vi "runnerFrontEnd.vi"(6 "ExperimentControlEvents":refnum<class "ExperimentControlEvents.lvclass">, 8 "error in (no error)":errorcluster, 9 "deviceDataBase":refnum<class "deviceDataBase.lvclass">, 10 "HWControllerEvents":refnum<class "HWControllerEvents.lvclass">, 11 "Views.lvlib:ExperimentControl.lvlib:ExperimentRunner in":refnum<class "ExperimentRunner.lvclass">) -> (0 "error out":errorcluster, 3 "Views.lvlib:ExperimentControl.lvlib:ExperimentRunner out":refnum<class "ExperimentRunner.lvclass">)   [LabVIEW 2011, in "Views.lvlib" / "ExperimentControl.lvlib" / "ExperimentRunner.lvclass"]
doc: "Experiment Runner Front End.\n\nThis is the user interface to control the expeirment. I.e. Run scripts and control the hardware state."
uses:
  ExperimentRunner.lvclass
  Hal/HWController/HWControllerEvents/HWControllerEvents.lvclass
  Tools/DatabaseHelpers/DbConnection/DeviceDataBase/deviceDataBase.lvclass
  Events/ExperimentControlEvents.lvclass
  ExperimentRunner.lvclass/ExperimentRunner.ctl
  CameraControlViewer/CameraControlViewer.lvclass
  Tools/SettingsProcessors/Compiler/Compiler.lvclass
  ScriptEditor/ScriptEditorV2/ScriptEditorV2.lvclass
  EventEditor/StaticOutputEditor/StaticOutputEditor.lvclass
  ScriptEditor/ScriptEdEvents/ScriptEdEvents.lvclass
  Tools/Filing/FileNeologist/FileNeologist.lvclass
  <vilib>/Utility/error.llb/DialogType.ctl
  Tools/DatabaseHelpers.lvlib
  Tools/Filing.lvlib
panel:
  in  "experimentFunction":enum16{"runListOnce", "loopOverList"}(ring)
  out "runningScriptName":string
  in  "HW Loop?":bool
  in  "refreshDatabase":bool
  in  "staticOutput":bool
  in  "stop":bool
  in  "runScript":bool
  in  "viewScript":bool
  in  "removePath":bool
  in  "addPath":bool
  out "status":T1(ring)
  in  "Listbox":i32(listbox)
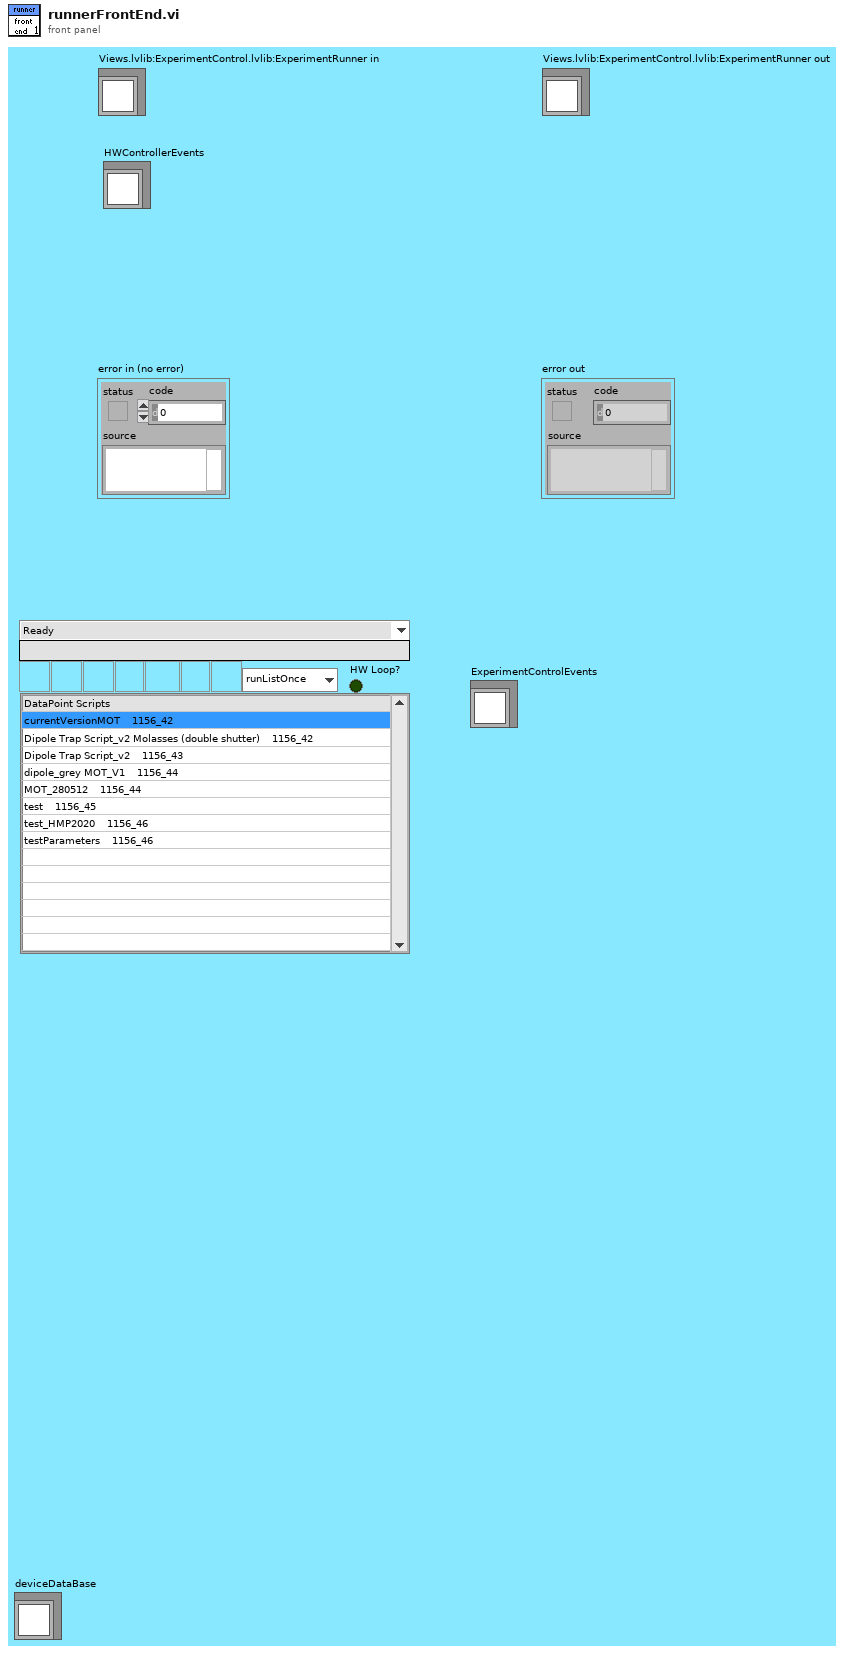
[diagram p1: front panel]
types:
  T1 = enum16{"Ready", "Compiling", "Configured", "Running", "Stopping", "Unresolved Error"}
  T2 = enum16{"start", "stop", "statusInquiry", "configure", "resetError", "resourcesInquiry", "reserveResources", "initialise", "resetAllChannels", "staticUpdate", "close", "HWStatus", "error", "resourcesAvailable", "resourcesReserved", "compilerError", "compiledScript", "compilingScript", "runScript", "configureCompiledScript"}
  T3 = enum16{"start", "stop", "statusInquiry", "configure", "resetError", "resourcesInquiry", "reserveResources", "initialise", "resetAllChannels", "staticUpdate", "close", "HWStatus", "error", "resourcesAvailable", "resourcesReserved"}
  T4 = enum16{"start", "stop", "statusInquiry", "configure", "resetError", "resourcesInquiry", "reserveResources", "initialise", "resetAllChannels", "staticUpdate", "close", "HWStatus", "error", "resourcesAvailable", "resourcesReserved", "compilerError", "compiledScript", "compilingScript", "runScript", "configureCompiledScript", "restartCompiler"}
  T5 = cluster{"incomingEventTypes":cluster{"start":cluster{"Boolean":bool}, "stop":cluster{"Boolean":bool}, "statusInquiry":cluster{"Boolean":bool}, "configure":cluster{"DPScriptPath":path, "TimeStamp":string, "HWLoop?":bool}, "resetError":cluster{"Boolean":bool}, "resourcesInquiry":cluster{"Boolean":bool}, "reserveResources":cluster{"HWList":string[]}, "initialise":cluster{"HWList":string[]}, "close":cluster{"Boolean":bool}, "resetAllChannels":cluster{"Boolean":bool}, "staticChannelUpdate":cluster{"channel_address":string, "calibratedValue":dbl}, "runScript":cluster{"DPScriptPath":path, "TimeStamp":string, "HWLoop?":bool}, "compilingScript":cluster{"Path":path}, "compiledScript":cluster{"Path":path, "timeCompileAt":string}, "compilerError":cluster{"Path":path}, "configureCompiledScript":cluster{"DPScriptPath":path, "TimeStamp":string, "HWLoop?":bool, "CompiledScript":cluster{"ScriptListCompiler.lvclass":refnum<class "ScriptListCompiler.lvclass">, "aoChannels":refnum<class "AnalogOutput.lvclass">[], "doChannels":refnum<class "DigitalOutput.lvclass">[], "rfChannels":refnum<class "DDSOutput.lvclass">[]}}, "restartCompiler":cluster{"restart":bool}, "staticRfChannelUpdate":cluster{"channel_address":string, "Output":cluster{"Frequency(MHz)":dbl, "Amplitude":dbl, "Phase":dbl, "OutputForm":enum16{"Sine", "Square", "Triangle", "Arbitrary"}}}, "cameraUpdate":cluster{"Camera":string, "Type":string, "settings":path}}, "outgoingEventTypes":cluster{"HWStatus":cluster{"status":enum16{"Ready", "Compiling", "Configured", "Running", "Stopping", "Unresolved Error"}}, "error":cluster{"error out":errorcluster}, "resourcesAvailable":cluster{"availableHWList":string[], "reservedHWList":string[]}, "resourcesReserved":cluster{"reservedHWList":string[]}}}
  T6 = cluster{"open":cluster{"Path":path}, "close":cluster{"Boolean":bool}, "save":cluster{"Path":path}}
  T7 = cluster{"eventId":enum16{"Open", "Save", "Close"}, "close":cluster{"Boolean":bool}}
  T8 = cluster{"eventId":enum16{"start", "stop", "statusInquiry", "configure", "resetError", "resourcesInquiry", "reserveResources", "initialise", "resetAllChannels", "staticUpdate", "close", "HWStatus", "error", "resourcesAvailable", "resourcesReserved", "compilerError", "compiledScript", "compilingScript", "runScript", "configureCompiledScript"}, cluster{bool}}
  T9 = cluster{"eventId":enum16{"Open", "Save", "Close"}, "open":cluster{"Path":path}}
  T10 = typedef "eventsource.ctl" = u32
  T11 = enum16{"start", "stop", "statusInquiry", "configure", "resetError", "resourcesInquiry", "reserveResources", "initialise", "resetAllChannels", "staticUpdate", "close", "HWStatus", "error", "resourcesAvailable", "resourcesReserved", "compilerError", "compiledScript", "compilingScript", "runScript", "configureCompiledScript", "restartCompiler", "staticRfChannelUpdate", "cameraUpdate"}
  T12 = cluster{"status":enum16{"Ready", "Compiling", "Configured", "Running", "Stopping", "Unresolved Error"}}
  T13 = typedef "DialogType.ctl" = u16
  T14 = cluster{"eventId":enum16{"start", "stop", "statusInquiry", "configure", "resetError", "resourcesInquiry", "reserveResources", "initialise", "resetAllChannels", "staticUpdate", "close", "HWStatus", "error", "resourcesAvailable", "resourcesReserved"}, "resetError":cluster{"Boolean":bool}}
  T15 = cluster{"eventId":enum16{"start", "stop", "statusInquiry", "configure", "resetError", "resourcesInquiry", "reserveResources", "initialise", "resetAllChannels", "staticUpdate", "close", "HWStatus", "error", "resourcesAvailable", "resourcesReserved"}, cluster{bool}}
  T16 = typedef "LVPoint32TypeDef.ctl" = cluster{"Horizontal":i32, "Vertical":i32}
  T17 = cluster{"eventId":enum16{"start", "stop", "statusInquiry", "configure", "resetError", "resourcesInquiry", "reserveResources", "initialise", "resetAllChannels", "staticUpdate", "close", "HWStatus", "error", "resourcesAvailable", "resourcesReserved", "compilerError", "compiledScript", "compilingScript", "runScript", "configureCompiledScript", "restartCompiler"}, cluster{bool}}
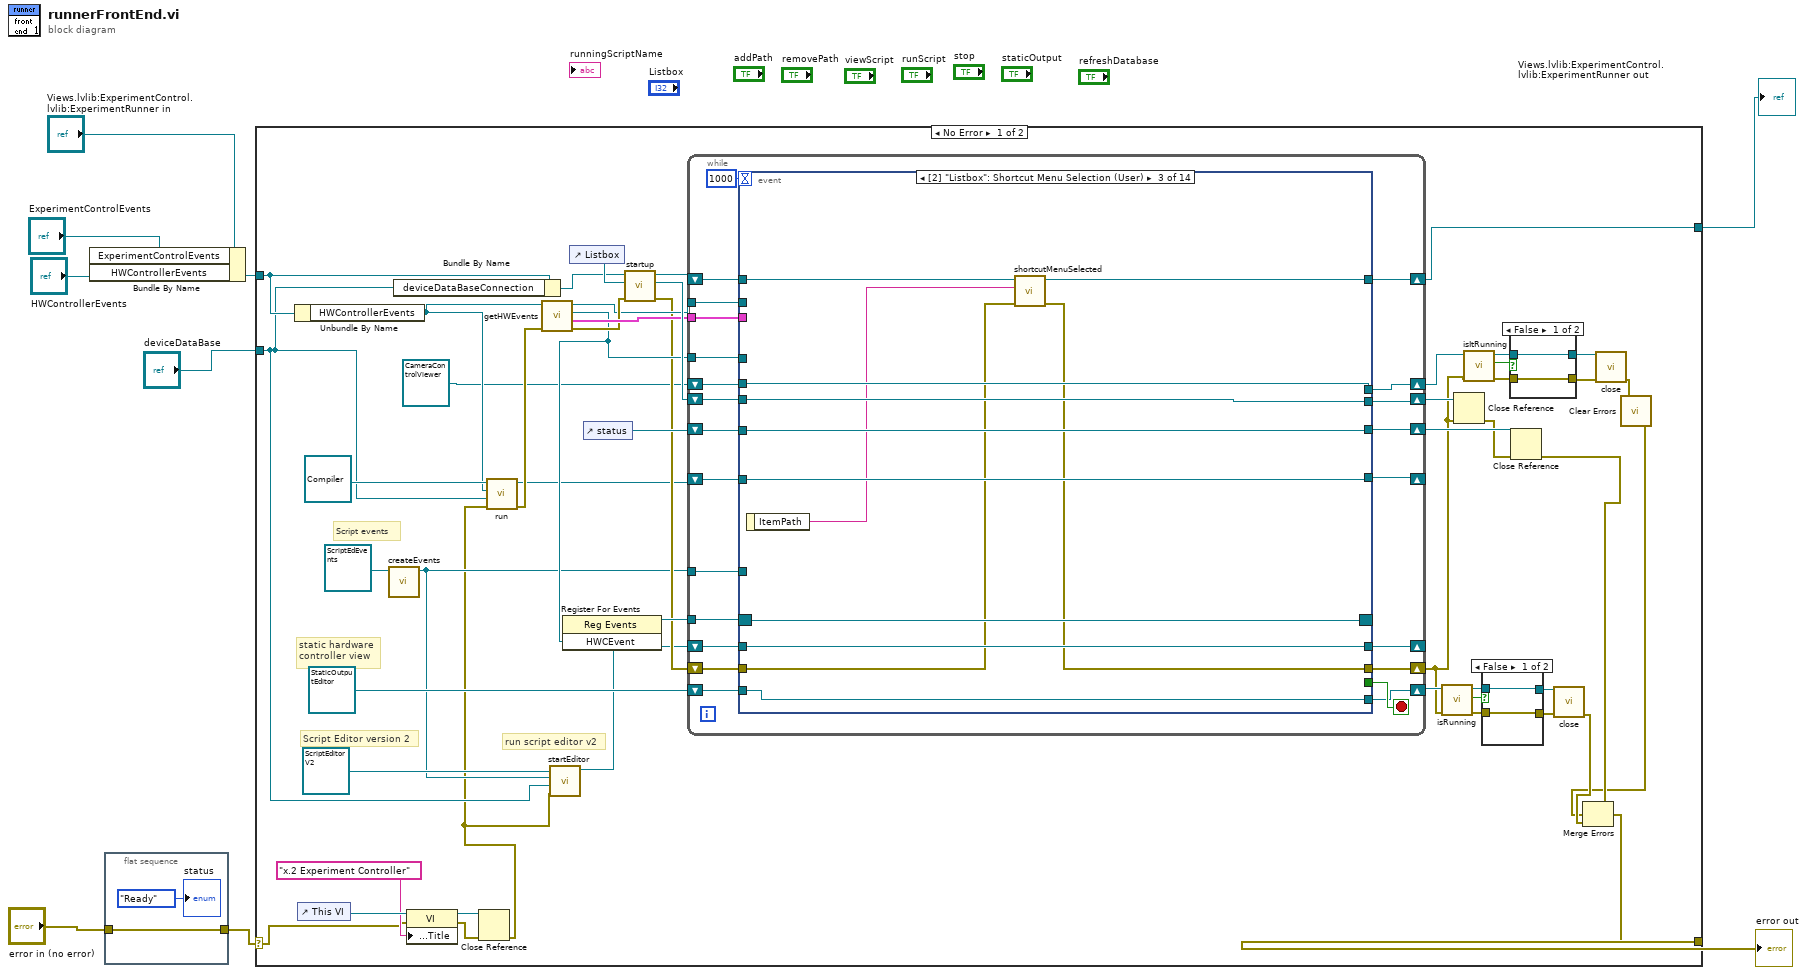
[diagram p0: block diagram]
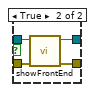
[diagram p2: hidden frame]
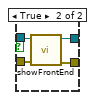
[diagram p3: hidden frame]
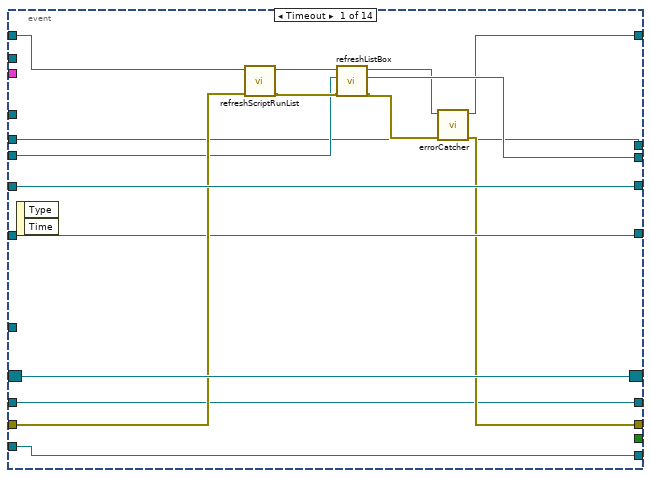
[diagram p4: hidden frame]
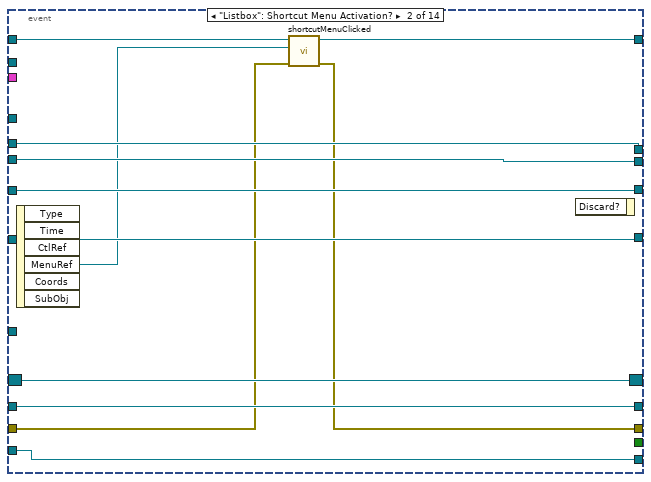
[diagram p5: hidden frame]
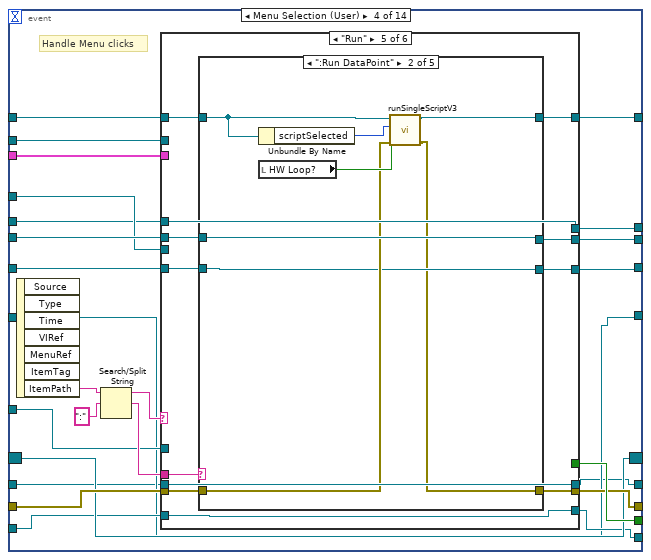
[diagram p6: hidden frame]
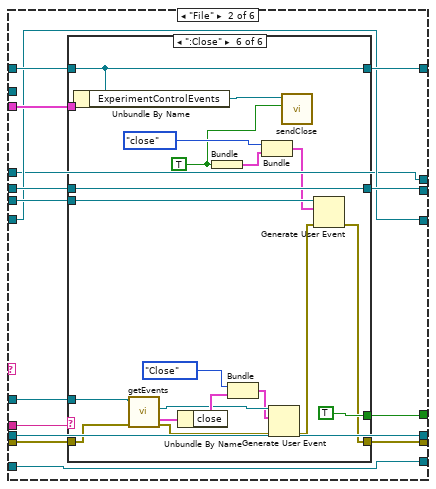
[diagram p8: hidden frame]
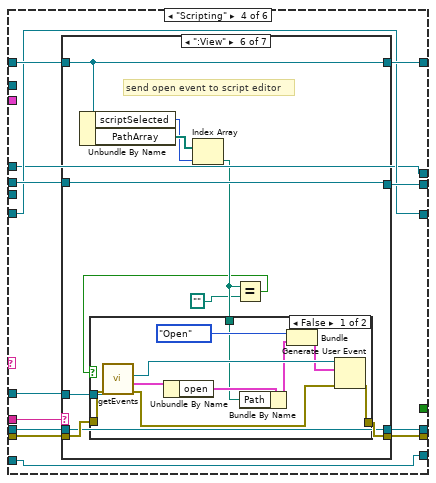
[diagram p20: hidden frame]
diagram:
  n1 = Bundle By Name(cluster="Views.lvlib:ExperimentControl.lvlib:ExperimentRunner in", "ExperimentControlEvents"="ExperimentControlEvents", "HWControllerEvents"="HWControllerEvents") -> (w5:refnum<class "ExperimentRunner.lvclass">)
  n2 = flat-sequence {
    tunnel: "error in (no error)" -> [w10]
    tunnel: [w10] -> w2
    frame #0 {
      "status" <- T1."Ready" ("status")
    }
  }
  n3 = case shown="No Error" w2 {
    selector: w2 -> [w37 w768]
    tunnel: [w50 w768] -> w9
    tunnel: [w41 w767] -> w8
    tunnel: w5 -> [w45 w767]
    tunnel: "deviceDataBase" -> [w25 _]
    frame No Error {
      # "run script editor v2"
      # "Script Editor version 2"
      # "Script events"
      # "static hardware\ncontroller view"
      n4 = Unbundle By Name(w45) -> ("HWControllerEvents"=w38:refnum<class "HWControllerEvents.lvclass">)
      n5 = control-ref of="This VI"() -> (w49:refnum<vi>)
      n6 = call-dynamic "createEvents.vi"("ScriptEdEvents in"=refnum<class "ScriptEdEvents.lvclass"> refnum ("Views.lvlib:SciptEditor.lvlib:ScriptEdEvents.lvclass")) -> ("ScriptEdEvents out"=w26:refnum<class "ScriptEdEvents.lvclass">)  [unwired: 9 in, 1 out]
      n7 = Bundle By Name(cluster=w45, "deviceDataBaseConnection"=w25) -> (w44:refnum<class "ExperimentRunner.lvclass">)
      n8 = property class="VI"(reference=w49, error in=w37, "Front Panel.Title"="x.2 Experiment Controller") -> (reference out=w47:refnum<vi>, error out=w46:errorcluster)
      n9 = Close Reference(reference=w47, error in (no error)=w46) -> (error out=w24:errorcluster)
      n10 = call "run.vi"("error in (no error)"=w24, "deviceDataBase"=w25, "HWControllerEvents"=w38, "Compiler in"=refnum<class "Compiler.lvclass"> refnum) -> ("error out"=w36:errorcluster, "Compiler out"=w35:refnum<class "Compiler.lvclass">)  [unwired: 6 in]
      n11 = call-dynamic "getHWEvents.vi"("error in (no error)"=w36, "HWControllerEvents in"=w38) -> ("error out"=w56:errorcluster, "eventDataTypes"=w57:T5, "HWCEvent"=w55:refnum<user-event>, "HWControllerEvents out"=w43:refnum<class "HWControllerEvents.lvclass">)  [unwired: 6 in]
      n12 = call "startEditor.vi"("error in (no error)"=w24, "deviceDataBase"=w25, "ScriptEdEvents"=w26, "ScriptEditorV2 in"=refnum<class "ScriptEditorV2.lvclass"> refnum ("Views.lvlib:SciptEditor.lvlib:ScriptEditorV2.lvclass")) -> ("ScriptEditorV2 out"=w23:refnum<class "ScriptEditorV2.lvclass">)  [unwired: 6 in, 1 out]
      n13 = register-events(w55) -> (reference out=w58:refnum<event-registration>)  [unwired: 2 in, 1 out]
      n14 = control-ref of="Listbox"() -> (w60:refnum<vi>)
      n15 = control-ref of="status"() -> (w54:refnum<vi>)
      n16 = call "startup.vi"("error in (no error)"=w56, "Listbox in"=w60, "ExperimentRunner in"=w44) -> ("error out"=w40:errorcluster, "Listbox out"=w59:refnum<vi>, "ExperimentRunner out"=w61:refnum<class "ExperimentRunner.lvclass">)  [unwired: 6 in]
      n17 = while {
        shift-right: [w96] -> w41
        shift-left: w61 -> [w83]
        shift-right: [w95] -> w19
        shift-left: w40 -> [w82]
        shift-right: [w94] -> w62
        shift-left: w59 -> [w84]
        tunnel: w58 -> [w93]
        tunnel: w57 -> [w92]
        tunnel: w55 -> [w91]
        shift-right: [w89] -> w53
        shift-left: w54 -> [w90]
        tunnel: w26 -> [w88]
        tunnel: w43 -> [w87]
        shift-right: [w85] -> w21
        shift-left: refnum<class "StaticOutputEditor.lvclass"> refnum ("Views.lvlib:SciptEditor.lvlib:StaticOutputEditor.lvclass") -> [w86]
        shift-right: [w79] -> _
        shift-left: w35 -> [w80]
        shift-right: [w78] -> _
        shift-left: w23 -> [w77]
        shift-right: [w75] -> w20
        shift-left: refnum<class "CameraControlViewer.lvclass"> refnum ("Views.lvlib:Camera.lvlib:CameraControlViewer.lvclass") -> [w76]
        stop <- w97 stop-if-true
        n18 = event shown="[2] \"Listbox\": Shortcut Menu Selection (User)" {
          selector: w93 -> [w112 w124 w136 w151 w460 _ _ w638 w652 w660 w695 w709 w718 w755]
          dyn-events: [w112 w124 w136 w151 w460 _ _ w638 w652 w660 w695 w709 w718 w755] -> _
          timeout: 1000 -> [_ _ _ _ _ _ _ _ _ _ _ _ _ _]
          tunnel: [_ _ _ w162 _ TRUE _ _ _ _ _ _ _ _] -> w97
          tunnel: w83 -> [w110 w118 w130 w157 w454 w590 w620 w642 w656 w672 w691 w703 w725 w765]
          tunnel: [w100 w114 w129 w156 w453 w589 w619 w636 w650 w672 w690 w702 w725 w764] -> w96
          tunnel: [w102 w115 w127 w154 w461 w594 w627 w632 w646 w668 w688 w704 w723 w744] -> w95
          tunnel: w82 -> [w109 w116 w128 w155 w462 w593 w616 w639 w654 w670 w692 w705 w715 w753]
          tunnel: w84 -> [w106 w119 w131 w153 w452 w610 w621 w635 w649 w671 w697 w708 w720 w762]
          tunnel: [w105 w119 w131 w152 w451 w610 w621 w634 w648 w671 w697 w708 w720 w762] -> w94
          tunnel: w92 -> [_ _ _ w150 w463 _ _ _ _ _ _ _ _ _]
          tunnel: w91 -> [_ _ _ w149 w456 w596 _ _ _ _ _ _ _ w759]
          tunnel: w90 -> [w113 w125 w137 w148 w459 w609 w617 w641 w655 w661 w689 w707 w719 w761]
          tunnel: [w113 w125 w137 w147 w458 w609 w617 w641 w655 w661 w689 w707 w719 w761] -> w89
          tunnel: w88 -> [_ _ _ w146 _ w595 _ _ _ w669 _ _ _ _]
          tunnel: w87 -> [_ _ _ w145 _ _ _ _ _ _ _ _ w724 _]
          tunnel: w86 -> [w111 w123 w135 w144 w455 w608 w615 w640 w653 w667 w696 w706 w710 w763]
          tunnel: [w111 w123 w135 w143 w455 w608 w615 w640 w653 w667 w696 w706 w722 w763] -> w85
          tunnel: w80 -> [w104 w122 w134 w142 w450 w587 w614 w631 w645 w659 w687 w700 w717 w748]
          tunnel: [w104 w122 w134 w142 w450 w587 w614 w631 w645 w659 w687 w700 w717 w745] -> w79
          tunnel: [w99 w121 w133 w140 w449 w586 w613 w630 w644 w658 w686 w699 w712 w743] -> w78
          tunnel: w77 -> [w99 w121 w133 w141 w449 w586 w613 w630 w644 w658 w686 w699 w712 w743]
          tunnel: w76 -> [w98 w120 w132 w139 w448 w585 w612 w629 w643 w657 w685 w698 w711 w742]
          tunnel: [w98 w120 w132 w138 w448 w585 w612 w629 w643 w657 w685 w698 w711 w742] -> w75
          event Timeout {
            n19 = event-data() -> ()  [unwired: 1 in, 2 out]
            n20 = call "refreshScriptRunList.vi"("error in (no error)"=w109, "ExperimentRunner in"=w110) -> ("error out"=w108:errorcluster, "ExperimentRunner out"=w107:refnum<class "ExperimentRunner.lvclass">)  [unwired: 8 in]
            n21 = call "refreshListBox.vi"("error in (no error)"=w108, "Listbox"=w106, "ExperimentRunner in"=w107) -> ("error out"=w103:errorcluster, "Listbox out"=w105:refnum<vi>, "ExperimentRunner out"=w101:refnum<class "ExperimentRunner.lvclass">)  [unwired: 6 in]
            n22 = call "errorCatcher.vi"("error in (no error)"=w103, "ExperimentRunner in"=w101) -> ("error out"=w102:errorcluster, "ExperimentRunner out"=w100:refnum<class "ExperimentRunner.lvclass">)  [unwired: 8 in]
          }
          event "Listbox": Shortcut Menu Activation? {
            n23 = event-data() -> ("MenuRef"=w117:refnum<k9>)  [unwired: 1 in, 5 out]
            n24 = call "shortcutMenuClicked.vi"("error in (no error)"=w116, "MenuRef"=w117, "ExperimentRunner in"=w118) -> ("error out"=w115:errorcluster, "ExperimentRunner out"=w114:refnum<class "ExperimentRunner.lvclass">)  [unwired: 7 in]
            n25 = event-data() -> ()  [unwired: 2 in, 1 out]
          }
          event "Listbox": Shortcut Menu Selection (User) {
            n26 = event-data() -> ("ItemPath"=w126:string)  [unwired: 1 in]
            n27 = call "shortcutMenuSelected.vi"("error in (no error)"=w128, "matlabScript"=w126, "ExperimentRunner in"=w130) -> ("error out"=w127:errorcluster, "ExperimentRunner out"=w129:refnum<class "ExperimentRunner.lvclass">)  [unwired: 7 in]
          }
          event Menu Selection (User) {
            # "Handle Menu clicks"
            n28 = event-data() -> ("ItemPath"=w160:string)  [unwired: 1 in, 6 out]
            n29 = Search/Split String(string=w160, search string/char (-)=":") -> (substring before match=w159:string, match + rest of string=w158:string)  [unwired: 1 in, 1 out]
            n30 = case shown="\"Run\"" w159 {
              tunnel: [_ w184 _ _ _ _] -> w162
              tunnel: w158 -> [_ w183 w225 w256 w348 w400]
              tunnel: w157 -> [w169 w182 w229 w260 w352 w399]
              tunnel: [w169 w181 w228 w259 w351 w398] -> w156
              tunnel: w155 -> [w168 w180 w226 w257 w349 w397]
              tunnel: [w168 w179 w227 w258 w350 w396] -> w154
              tunnel: w153 -> [w167 w178 w224 w255 w347 w395]
              tunnel: [w167 w177 w223 w254 w346 w395] -> w152
              tunnel: w150 -> [_ w176 _ _ _ _]
              tunnel: w149 -> [_ w175 _ _ _ w393]
              tunnel: w148 -> [w166 w174 w222 w253 w345 w394]
              tunnel: [w166 w174 w222 w253 w344 w394] -> w147
              tunnel: w146 -> [_ w173 _ w252 _ _]
              tunnel: w145 -> [_ _ _ _ _ w392]
              tunnel: w144 -> [w165 w172 w221 w251 w343 w391]
              tunnel: [w165 w172 w221 w251 w343 w390] -> w143
              tunnel: w141 -> [w164 w171 w220 w250 w342 w389]
              tunnel: [w164 w171 w220 w249 w342 w389] -> w140
              tunnel: w139 -> [w163 w170 w219 w248 w341 w388]
              tunnel: [w163 w170 w219 w248 w341 w387] -> w138
              frame "False", Default {
              }
              frame "File" {
                n31 = case shown="\":Close\"" w183 {
                  tunnel: [_ _ _ _ _ TRUE] -> w184
                  tunnel: [w187 w190 w193 w196 w199 w202] -> w181
                  tunnel: w182 -> [w187 w190 w193 w196 w199 w202]
                  tunnel: w180 -> [w186 w189 w192 w195 w198 w204]
                  tunnel: [w186 w189 w192 w195 w198 w213] -> w179
                  tunnel: w178 -> [w185 w188 w191 w194 w197 w217]
                  tunnel: [w185 w188 w191 w194 w197 w217] -> w177
                  tunnel: w176 -> [_ _ _ _ _ _]
                  tunnel: w175 -> [_ _ _ _ _ w216]
                  tunnel: w173 -> [_ _ _ _ _ w212]
                  frame Default {
                  }
                  frame ":Open" {
                  }
                  frame ":Load" {
                  }
                  frame ":Save" {
                  }
                  frame ":Save As" {
                  }
                  frame ":Close" {
                    w200 = TRUE
                    n32 = Unbundle By Name(w202) -> ("ExperimentControlEvents"=w201:refnum<class "ExperimentControlEvents.lvclass">)
                    n33 = call-dynamic "getEvents.vi"("error in (no error)"=w204, "ScriptEdEvents in"=w212) -> ("error out"=w206:errorcluster, "eventsToScriptEd"=w211:T6, "ScriptEvent"=w208:refnum<user-event>)  [unwired: 6 in, 1 out]
                    n34 = Unbundle By Name(w211) -> ("close"=w209:cluster{"Boolean":bool})
                    n35 = Bundle(w200) -> (w215:cluster{bool})  [unwired: 1 in]
                    n36 = Bundle("eventId"=enum16{"Open", "Save", "Close"}."Close", "close"=w209) -> (w207:T7)  [unwired: 1 in]
                    n37 = Bundle("eventId"=T2."close", w215) -> (w214:T8)  [unwired: 1 in]
                    n38 = Generate User Event(user event=w208, event data cluster=w207, error in=w206) -> (error out=w205:errorcluster)  [unwired: 1 out]
                    n39 = call "sendClose.vi"("close"=w200, "ExperimentControlEvents in"=w201) -> ()  [unwired: 8 in, 2 out]
                    n40 = Generate User Event(user event=w216, event data cluster=w214, error in=w205) -> (error out=w213:errorcluster)  [unwired: 1 out]
                  }
                }
              }
              frame "Edit" {
                n41 = case shown="\":Paste\"" w225 {
                  tunnel: [w232 w235 w238 w241 w244 w247] -> w228
                  tunnel: w229 -> [w232 w235 w238 w241 w244 w247]
                  tunnel: [w231 w234 w237 w240 w243 w246] -> w227
                  tunnel: w226 -> [w231 w234 w237 w240 w243 w246]
                  tunnel: w224 -> [w230 w233 w236 w239 w242 w245]
                  tunnel: [w230 w233 w236 w239 w242 w245] -> w223
                  frame Default {
                  }
                  frame ":Undo" {
                  }
                  frame ":Redo" {
                  }
                  frame ":Change Order" {
                  }
                  frame ":Copy" {
                  }
                  frame ":Paste" {
                  }
                }
              }
              frame "Scripting" {
                n42 = case shown="\":View\"" w256 {
                  tunnel: [w264 w269 w277 w287 w294 w308 w324] -> w259
                  tunnel: w260 -> [w264 w273 w282 w291 w298 w308 w324]
                  tunnel: [w263 w266 w279 w288 w293 w303 w326] -> w258
                  tunnel: w257 -> [w263 w272 w281 w290 w296 w304 w330]
                  tunnel: w255 -> [w262 w268 w276 w285 w297 w309 w332]
                  tunnel: [w262 w267 w275 w284 w295 w309 w332] -> w254
                  tunnel: w252 -> [_ _ _ _ _ w305 w322]
                  tunnel: w250 -> [w261 w265 w274 w283 w292 w299 w331]
                  tunnel: [w261 w265 w274 w283 w292 w299 w328] -> w249
                  frame Default {
                  }
                  frame ":Add" {
                    n43 = call "loadDPScript.vi"("error in (no error)"=w272, "ExperimentRunner in"=w273) -> ("error out"=w271:errorcluster, "ExperimentRunner out"=w270:refnum<class "ExperimentRunner.lvclass">)  [unwired: 8 in]
                    n44 = call "refreshListBox.vi"("error in (no error)"=w271, "Listbox"=w268, "ExperimentRunner in"=w270) -> ("error out"=w266:errorcluster, "Listbox out"=w267:refnum<vi>, "ExperimentRunner out"=w269:refnum<class "ExperimentRunner.lvclass">)  [unwired: 6 in]
                  }
                  frame ":Refresh" {
                    n45 = call "refreshScriptRunList.vi"("error in (no error)"=w281, "ExperimentRunner in"=w282) -> ("error out"=w280:errorcluster, "ExperimentRunner out"=w278:refnum<class "ExperimentRunner.lvclass">)  [unwired: 8 in]
                    n46 = call "refreshListBox.vi"("error in (no error)"=w280, "Listbox"=w276, "ExperimentRunner in"=w278) -> ("error out"=w279:errorcluster, "Listbox out"=w275:refnum<vi>, "ExperimentRunner out"=w277:refnum<class "ExperimentRunner.lvclass">)  [unwired: 6 in]
                  }
                  frame ":Remove" {
                    n47 = call "removeDPScript.vi"("error in (no error)"=w290, "ExperimentRunner in"=w291) -> ("error out"=w289:errorcluster, "ExperimentRunner out"=w286:refnum<class "ExperimentRunner.lvclass">)  [unwired: 8 in]
                    n48 = call "refreshListBox.vi"("error in (no error)"=w289, "Listbox"=w285, "ExperimentRunner in"=w286) -> ("error out"=w288:errorcluster, "Listbox out"=w284:refnum<vi>, "ExperimentRunner out"=w287:refnum<class "ExperimentRunner.lvclass">)  [unwired: 6 in]
                  }
                  frame ":Remove All" {
                    n49 = call "clearAllFromRun.vi"("error in (no error)"=w296, "Listbox in"=w297, "ExperimentRunner in"=w298) -> ("error out"=w293:errorcluster, "Listbox out"=w295:refnum<vi>, "ExperimentRunner out"=w294:refnum<class "ExperimentRunner.lvclass">)  [unwired: 6 in]
                  }
                  frame ":View" {
                    # "send open event to script editor"
                    n50 = Unbundle By Name(w308) -> ("scriptSelected"=w306:i32, "PathArray"=w307:path[])
                    n51 = Index Array(array=w307, index=w306) -> (element=w302:path)
                    n52 = Equal?(x=w302, y=path "") -> (x = y?=w300:bool)
                    n53 = case shown="False" w300 {
                      tunnel: w305 -> [w320 _]
                      tunnel: w304 -> [w319 w321]
                      tunnel: [w311 w321] -> w303
                      tunnel: w302 -> [w310 _]
                      frame False {
                        n54 = call-dynamic "getEvents.vi"("error in (no error)"=w319, "ScriptEdEvents in"=w320) -> ("error out"=w312:errorcluster, "eventsToScriptEd"=w318:T6, "ScriptEvent"=w316:refnum<user-event>)  [unwired: 6 in, 1 out]
                        n55 = Unbundle By Name(w318) -> ("open"=w317:cluster{"Path":path})
                        n56 = Bundle By Name(cluster=w317, "Path"=w310) -> (w314:cluster{"Path":path})
                        n57 = Bundle("eventId"=enum16{"Open", "Save", "Close"}."Open", "open"=w314) -> (w313:T9)  [unwired: 1 in]
                        n58 = Generate User Event(user event=w316, event data cluster=w313, error in=w312) -> (error out=w311:errorcluster)  [unwired: 1 out]
                      }
                      frame True {
                      }
                    }
                  }
                  frame ":Open Script Editor" {
                    n59 = Unbundle By Name(w324) -> ("deviceDataBaseConnection"=w323:refnum<class "deviceDataBase.lvclass">)
                    n60 = call "isRunning.vi"("error in (no error)"=w330, "ScriptEditorV2 in"=w331) -> ("error out"=w325:errorcluster, "Running?"=w329:bool, "ScriptEditorV2 out"=w327:refnum<class "ScriptEditorV2.lvclass">)  [unwired: 7 in]
                    n61 = case shown="False" w329 {
                      tunnel: [w336 w340] -> w328
                      tunnel: w327 -> [w338 w340]
                      tunnel: [w335 w339] -> w326
                      tunnel: w325 -> [w337 w339]
                      tunnel: w323 -> [w334 _]
                      tunnel: w322 -> [w333 _]
                      frame False {
                        n62 = call "startEditor.vi"("error in (no error)"=w337, "deviceDataBase"=w334, "ScriptEdEvents"=w333, "ScriptEditorV2 in"=w338) -> ("error out"=w335:errorcluster, "ScriptEditorV2 out"=w336:refnum<class "ScriptEditorV2.lvclass">)  [unwired: 6 in]
                      }
                      frame True {
                      }
                    }
                  }
                }
              }
              frame "Run" {
                n63 = case shown="\":Run DataPoint\"" w348 {
                  tunnel: [w356 w362 w369 w376 w383] -> w351
                  tunnel: w352 -> [w356 w363 w371 w377 w384]
                  tunnel: [w355 w357 w367 w374 w382] -> w350
                  tunnel: w349 -> [w355 w359 w368 w375 w381]
                  tunnel: w347 -> [w354 w364 w372 w379 w386]
                  tunnel: [w354 w364 w372 w379 w386] -> w346
                  tunnel: w345 -> [w353 w358 w366 w378 w385]
                  tunnel: [w353 w358 w366 w378 w385] -> w344
                  frame Default {
                  }
                  frame ":Run DataPoint" {
                    n64 = Unbundle By Name(w363) -> ("scriptSelected"=w361:i32)
                    n65 = local read "HW Loop?"() -> (w360:bool)
                    n66 = call "runSingleScriptV3.vi"("error in (no error)"=w359, "HWLoop"=w360, "index"=w361, "ExperimentRunner in"=w363) -> ("error out"=w357:errorcluster, "ExperimentRunner out"=w362:refnum<class "ExperimentRunner.lvclass">)  [unwired: 6 in]
                  }
                  frame ":Run Experiment" {
                    n67 = Unbundle By Name(w371) -> ("scriptSelected"=w370:i32)
                    n68 = call "runExperimentV2.vi"("error in (no error)"=w368, "runExperiment.Enum"="experimentFunction", "index"=w370, "ExperimentRunner in"=w371) -> ("error out"=w367:errorcluster, "ExperimentRunner out"=w369:refnum<class "ExperimentRunner.lvclass">)  [unwired: 6 in]
                  }
                  frame ":Pause Experiment" {
                    n69 = call "sendStop.vi"("error in (no error)"=w375, "stop"=enum16{"stopBeforeNext", "stopNow"}."stopBeforeNext", "ExperimentRunner in"=w377) -> ("error out"=w374:errorcluster, "ExperimentRunner out"=w376:refnum<class "ExperimentRunner.lvclass">)  [unwired: 7 in]
                  }
                  frame ":Stop" {
                    n70 = call "sendStop.vi"("error in (no error)"=w381, "stop"=enum16{"stopBeforeNext", "stopNow"}."stopNow", "ExperimentRunner in"=w384) -> ("error out"=w382:errorcluster, "ExperimentRunner out"=w383:refnum<class "ExperimentRunner.lvclass">)  [unwired: 7 in]
                  }
                }
              }
              frame "Hardware Control" {
                n71 = case shown="\":Camera Control\"" w400 {
                  tunnel: w399 -> [w404 w415 w439]
                  tunnel: [w404 w415 w439] -> w398
                  tunnel: w397 -> [w403 w408 w434]
                  tunnel: [w403 w412 w438] -> w396
                  tunnel: w393 -> [_ _ _]
                  tunnel: w392 -> [_ w414 _]
                  tunnel: w391 -> [w402 w405 w431]
                  tunnel: [w402 w413 w431] -> w390
                  tunnel: w388 -> [w401 w406 w433]
                  tunnel: [w401 w406 w432] -> w387
                  frame "False", Default {
                  }
                  frame ":Update Channel Output" {
                    n72 = Unbundle By Name(w415) -> ("deviceDataBaseConnection"=w411:refnum<class "deviceDataBase.lvclass">)
                    n73 = call "isRunning.vi"("error in (no error)"=w408, "StaticOutputEditor in"=w405) -> ("error out"=w409:errorcluster, "running?"=w407:bool, "StaticOutputEditor out"=w410:refnum<class "StaticOutputEditor.lvclass">)  [unwired: 7 in]
                    n74 = case shown="False" w407 {
                      tunnel: w410 -> [w426 w430]
                      tunnel: w414 -> [w424 _]
                      tunnel: [w423 w428] -> w413
                      tunnel: [w422 w427] -> w412
                      tunnel: w411 -> [w421 _]
                      tunnel: w409 -> [w419 w429]
                      frame False {
                        n75 = call "close.vi"("error in (no error)"=w419, "StaticOutputEditor in"=w426) -> ("error out"=w418:errorcluster, "StaticOutputEditor out"=w425:refnum<class "StaticOutputEditor.lvclass">)  [unwired: 8 in]
                        n76 = call "getUnrestrictedChannelArray.vi"("error in (no error)"=w419, "deviceDataBase in"=w421) -> ("error out"=w417:errorcluster, "ChannelArray.lvclass"=w420:refnum<class "ChannelArray.lvclass">)  [unwired: 7 in, 1 out]
                        n77 = Merge Errors(w418, w417) -> (w416:errorcluster)
                        n78 = call-dynamic "run.vi"("error in (no error)"=w416, "HWControllerEvents"=w424, "ChannelArray"=w420, "StaticOutputEditor"=w425) -> ("error out"=w422:errorcluster, "StaticOutputEditor out"=w423:refnum<class "StaticOutputEditor.lvclass">)  [unwired: 6 in]
                      }
                      frame True {
                        n79 = call "showFrontEnd.vi"("error in (no error)"=w429, "StaticOutputEditor in"=w430) -> ("error out"=w427:errorcluster, "StaticOutputEditor out"=w428:refnum<class "StaticOutputEditor.lvclass">)  [unwired: 8 in]
                      }
                    }
                  }
                  frame ":Camera Control" {
                    n80 = call "isItRunning.vi"("error in (no error)"=w434, "CameraControlViewer in"=w433) -> ("error out"=w437:errorcluster, "running?"=w435:bool, "CameraControlViewer out"=w436:refnum<class "CameraControlViewer.lvclass">)  [unwired: 7 in]
                    n81 = case shown="False" w435 {
                      tunnel: w436 -> [w441 w445]
                      tunnel: [w443 w446] -> w438
                      tunnel: w437 -> [w440 w447]
                      tunnel: [w442 w444] -> w432
                      frame False {
                        n82 = call "launch.vi"("error in (no error)"=w440, "CameraControlViewer in"=w441) -> ("error out"=w443:errorcluster, "CameraControlViewer out"=w442:refnum<class "CameraControlViewer.lvclass">)  [unwired: 8 in]
                      }
                      frame True {
                        n83 = call "showFrontEnd.vi"("error in (no error)"=w447, "CameraControlViewer in"=w445) -> ("error out"=w446:errorcluster, "CameraControlViewer out"=w444:refnum<class "CameraControlViewer.lvclass">)  [unwired: 8 in]
                      }
                    }
                  }
                }
              }
            }
          }
          event User Event {
            # "recieve hardware events."
            n84 = event-data() -> ("Source"=w457:T10, "eventId"=w465:T11, "data"=w464:variant)  [unwired: 1 in, 3 out]
            n85 = case shown="\"HWStatus\"" w465 {
              tunnel: w464 -> [_ w481 w492 w522 w537 w572 _ _]
              tunnel: w463 -> [_ w480 w499 w531 w545 w570 _ _]
              tunnel: w462 -> [w468 w478 w491 w517 w533 w571 w580 w584]
              tunnel: [w468 w473 w496 w528 w542 w558 w580 w584] -> w461
              tunnel: w459 -> [w469 w475 w493 w525 w539 w567 w579 w583]
              tunnel: [w469 w474 w493 w525 w539 w565 w579 w583] -> w458
              tunnel: w457 -> [_ _ _ _ _ _ _ _]
              tunnel: w456 -> [_ _ _ _ _ w564 _ _]
              tunnel: w454 -> [w467 w472 w498 w530 w544 w548 w578 w582]
              tunnel: [w467 w472 w497 w529 w543 w548 w578 w582] -> w453
              tunnel: w452 -> [w466 w471 w495 w527 w541 w547 w577 w581]
              tunnel: [w466 w471 w494 w526 w540 w547 w577 w581] -> w451
              frame Default {
              }
              frame "HWStatus" {
                n86 = Unbundle By Name(w480) -> ("outgoingEventTypes.HWStatus"=w479:T12)
                n87 = Variant To Data(error in=w478, type=w479, Variant=w481) -> (data=w476:T12, error out=w477:errorcluster)
                n88 = Unbundle By Name(w476) -> ("status"=w470:T1)
                n89 = case shown="\"Running\"" w470 {
                  frame "Ready", Default {
                    n90 = local write "runningScriptName"("") -> ()
                  }
                  frame "Unresolved Error" {
                    n91 = local write "runningScriptName"("") -> ()
                  }
                  frame "Running" {
                    n92 = call "globalFileNeologist.vi"("Action"=enum16{"Write", "Read"}."Read") -> ("FileNeologist out"=w489:refnum<class "FileNeologist.lvclass">)  [unwired: 10 in]
                    n93 = call <vilib>:"Space Constant.vi"() -> ("String"=w485:string)
                    n94 = call-dynamic "getScriptName.vi"("FileNeologist.lvclass in"=w489) -> ("scriptName"=w486:string, "FileNeologist.lvclass out"=w488:refnum<class "FileNeologist.lvclass">)  [unwired: 8 in, 1 out]
                    n95 = call "getTimeStamp.vi"("FileNeologist in"=w488) -> ("TimeStamp"=w487:string)  [unwired: 8 in, 2 out]
                    n96 = Concatenate Strings(w487, w485, w486) -> (w484:string)
                    n97 = local write "runningScriptName"(w484) -> ()
                  }
                  frame "Stopping" {
                  }
                  frame "Configured" {
                  }
                }
                n98 = property class="Enum (strict)"(reference=w475, error in=w477, "Value"=w470) -> (reference out=w474:refnum<vi>, error out=w473:errorcluster)
              }
              frame "compilerError" {
                n99 = disable-structure shown="Enabled" {
                  disable-tunnel: w499 -> [w512 _]
                  disable-tunnel: w498 -> [w511 w515]
                  disable-tunnel: [w510 w515] -> w497
                  disable-tunnel: [w509 w513] -> w496
                  disable-tunnel: w495 -> [w508 w514]
                  disable-tunnel: [w507 w514] -> w494
                  disable-tunnel: w492 -> [w505 _]
                  disable-tunnel: w491 -> [w501 w513]
                  frame Disabled {
                    n100 = Unbundle By Name(w512) -> ("incomingEventTypes.compilerError"=w504:cluster{"Path":path})
                    n101 = Variant To Data(error in=w501, type=w504, Variant=w505) -> (data=w503:cluster{"Path":path}, error out=w500:errorcluster)
                    n102 = Unbundle By Name(w503) -> ("Path"=w502:path)
                    n103 = call "compilerUpdate.vi"("String"="    Compiler Error", "error in (no error)"=w500, "Path"=w502, "Listbox in"=w508, "ExperimentRunner in"=w511) -> ("error out"=w509:errorcluster, "Listbox out"=w507:refnum<vi>, "ExperimentRunner out"=w510:refnum<class "ExperimentRunner.lvclass">)  [unwired: 4 in]
                  }
                  frame Enabled {
                  }
                }
              }
              frame "compiledScript" {
                n104 = Unbundle By Name(w531) -> ("incomingEventTypes.compiledScript"=w521:cluster{"Path":path, "timeCompileAt":string})
                n105 = Variant To Data(error in=w517, type=w521, Variant=w522) -> (data=w520:cluster{"Path":path, "timeCompileAt":string}, error out=w516:errorcluster)
                n106 = Unbundle By Name(w520) -> ("timeCompileAt"=w519:string, "Path"=w518:path)
                n107 = Concatenate Strings("    ", w519) -> (w523:string)
                n108 = call "compilerUpdate.vi"("String"=w523, "error in (no error)"=w516, "Path"=w518, "Listbox in"=w527, "ExperimentRunner in"=w530) -> ("error out"=w528:errorcluster, "Listbox out"=w526:refnum<vi>, "ExperimentRunner out"=w529:refnum<class "ExperimentRunner.lvclass">)  [unwired: 4 in]
              }
              frame "compilingScript" {
                n109 = Unbundle By Name(w545) -> ("incomingEventTypes.compilingScript"=w536:cluster{"Path":path})
                n110 = Variant To Data(error in=w533, type=w536, Variant=w537) -> (data=w534:cluster{"Path":path}, error out=w532:errorcluster)
                n111 = Unbundle By Name(w534) -> ("Path"=w535:path)
                n112 = call "compilerUpdate.vi"("String"="    Compiling", "error in (no error)"=w532, "Path"=w535, "Listbox in"=w541, "ExperimentRunner in"=w544) -> ("error out"=w542:errorcluster, "Listbox out"=w540:refnum<vi>, "ExperimentRunner out"=w543:refnum<class "ExperimentRunner.lvclass">)  [unwired: 4 in]
              }
              frame "error" {
                w546 = T13 1 items=["no dialog", "OK message", "continue or stop message", "OK message + warnings", "continue/stop + warnings"] ("type of dialog (OK msg:1)")
                w553 = "\r\n"
                n113 = Unbundle By Name(w570) -> ("incomingEventTypes.resetError"=w563:cluster{"Boolean":bool}, "outgoingEventTypes.error"=w569:cluster{"error out":errorcluster})
                n114 = Variant To Data(error in=w571, type=w569, Variant=w572) -> (data=w568:cluster{"error out":errorcluster}, error out=w566:errorcluster)
                n115 = Unbundle By Name(w568) -> ("error out"=w555:errorcluster)
                n116 = Bundle By Name(cluster=w563, "Boolean"=TRUE) -> (w561:cluster{"Boolean":bool})
                n117 = Unbundle By Name(w555) -> ("source"=w552:string)
                n118 = property class="Enum (strict)"(reference=w567, error in=w566, "Value"=T1."Unresolved Error") -> (reference out=w565:refnum<vi>, error out=w559:errorcluster)
                n119 = Bundle("eventId"=T3."resetError", "resetError"=w561) -> (w560:T14)  [unwired: 1 in]
                n120 = Concatenate Strings(w552, w553, w553, "\nA hardware error has occured with the above code. Clicking ok will clear the error, however restarting the program or labview may be necessary depending on the problem.") -> (w556:string)
                n121 = Bundle By Name(cluster=w555, "source"=w556) -> (w554:errorcluster)
                n122 = flat-sequence {
                  tunnel: w564 -> [w576]
                  tunnel: w560 -> [w575]
                  tunnel: w559 -> [w574]
                  tunnel: [w573] -> w558
                  tunnel: w557 -> [_]
                  frame #0 {
                    n123 = Generate User Event(user event=w576, event data cluster=w575, error in=w574) -> (error out=w573:errorcluster)  [unwired: 1 out]
                  }
                }
                n124 = call <vilib>:"Simple Error Handler.vi"("type of dialog (OK msg:1)"=w546, "error in (no error)"=w554) -> ("error out"=w557:errorcluster)  [unwired: 3 in, 4 out]
              }
              frame "resourcesAvailable" {
              }
              frame "resourcesReserved" {
              }
            }
          }
          event Panel Close {
            # "close"
            n125 = event-data() -> ()  [unwired: 1 in, 4 out]
            n126 = Unbundle By Name(w590) -> ("ExperimentControlEvents"=w592:refnum<class "ExperimentControlEvents.lvclass">)
            n127 = call-dynamic "getEvents.vi"("error in (no error)"=w593, "ScriptEdEvents in"=w595) -> ("error out"=w599:errorcluster, "eventsToScriptEd"=w604:T6, "ScriptEvent"=w601:refnum<user-event>)  [unwired: 6 in, 1 out]
            n128 = Unbundle By Name(w604) -> ("close"=w602:cluster{"Boolean":bool})
            n129 = Bundle(TRUE) -> (w606:cluster{bool})  [unwired: 1 in]
            n130 = call "sendClose.vi"("close"=TRUE, "ExperimentControlEvents in"=w592) -> ("ExperimentControlEvents out"=w588:refnum<class "ExperimentControlEvents.lvclass">)  [unwired: 8 in, 1 out]
            n131 = Bundle("eventId"=enum16{"Open", "Save", "Close"}."Close", "close"=w602) -> (w600:T7)  [unwired: 1 in]
            n132 = Bundle("eventId"=T3."close", w606) -> (w605:T15)  [unwired: 1 in]
            n133 = Generate User Event(user event=w601, event data cluster=w600, error in=w599) -> (error out=w598:errorcluster)  [unwired: 1 out]
            n134 = Bundle By Name(cluster=w590, "ExperimentControlEvents"=w588) -> (w589:refnum<class "ExperimentRunner.lvclass">)
            n135 = Generate User Event(user event=w596, event data cluster=w605, error in=w598) -> (error out=w594:errorcluster)  [unwired: 1 out]
          }
          event "Listbox": Mouse Down {
            # "select row of listbox"
            n136 = event-data() -> ("CtlRef"=w622:refnum<vi>, "Coords"=w628:T16)  [unwired: 1 in, 6 out]
            n137 = invoke class="LstBox (strict)" method="Point To Row"(reference=w622, error in=w616, "Point"=w628) -> (reference out=w626:refnum<vi>, error out=w625:errorcluster, "Row"=w618:i32)  [unwired: 4 in, 4 out]
            n138 = property class="LstBox (strict)"(reference=w626, error in=w625, "Value"=w618) -> (reference out=w623:refnum<vi>, error out=w624:errorcluster)
            n139 = Bundle By Name(cluster=w620, "scriptSelected"=w618) -> (w619:refnum<class "ExperimentRunner.lvclass">)
            n140 = Close Reference(reference=w623, error in (no error)=w624) -> (error out=w627:errorcluster)
          }
          event "addPath": Mouse Down {
            # "ADD A PATH"
            n141 = event-data() -> ()  [unwired: 1 in, 8 out]
            n142 = call "loadDPScript.vi"("error in (no error)"=w639, "ExperimentRunner in"=w642) -> ("error out"=w633:errorcluster, "ExperimentRunner out"=w637:refnum<class "ExperimentRunner.lvclass">)  [unwired: 8 in]
            n143 = call "refreshListBox.vi"("error in (no error)"=w633, "Listbox"=w635, "ExperimentRunner in"=w637) -> ("error out"=w632:errorcluster, "Listbox out"=w634:refnum<vi>, "ExperimentRunner out"=w636:refnum<class "ExperimentRunner.lvclass">)  [unwired: 6 in]
          }
          event "removePath": Mouse Down {
            n144 = event-data() -> ()  [unwired: 1 in, 8 out]
            n145 = call "removeDPScript.vi"("error in (no error)"=w654, "ExperimentRunner in"=w656) -> ("error out"=w647:errorcluster, "ExperimentRunner out"=w651:refnum<class "ExperimentRunner.lvclass">)  [unwired: 8 in]
            n146 = call "refreshListBox.vi"("error in (no error)"=w647, "Listbox"=w649, "ExperimentRunner in"=w651) -> ("error out"=w646:errorcluster, "Listbox out"=w648:refnum<vi>, "ExperimentRunner out"=w650:refnum<class "ExperimentRunner.lvclass">)  [unwired: 6 in]
          }
          event "viewScript": Mouse Down {
            # "send nothing is blank path"
            # "open a script in script editor.\nby sending an open event with the path\nof the script."
            n147 = event-data() -> ()  [unwired: 1 in, 8 out]
            n148 = Unbundle By Name(w672) -> ("scriptSelected"=w665:i32, "PathArray"=w666:path[])
            n149 = Index Array(array=w666, index=w665) -> (element=w664:path)
            n150 = Equal?(x=w664, y=path "") -> (x = y?=w662:bool)
            n151 = case shown="False" w662 {
              tunnel: w669 -> [w683 _]
              tunnel: w670 -> [w682 w684]
              tunnel: [w674 w684] -> w668
              tunnel: w664 -> [w673 _]
              frame False {
                n152 = call-dynamic "getEvents.vi"("error in (no error)"=w682, "ScriptEdEvents in"=w683) -> ("error out"=w675:errorcluster, "eventsToScriptEd"=w681:T6, "ScriptEvent"=w679:refnum<user-event>)  [unwired: 6 in, 1 out]
                n153 = Unbundle By Name(w681) -> ("open"=w680:cluster{"Path":path})
                n154 = Bundle By Name(cluster=w680, "Path"=w673) -> (w677:cluster{"Path":path})
                n155 = Bundle("eventId"=enum16{"Open", "Save", "Close"}."Open", "open"=w677) -> (w676:T9)  [unwired: 1 in]
                n156 = Generate User Event(user event=w679, event data cluster=w676, error in=w675) -> (error out=w674:errorcluster)  [unwired: 1 out]
              }
              frame True {
              }
            }
          }
          event "runScript": Mouse Down {
            # "Run a Single Script"
            n157 = event-data() -> ()  [unwired: 1 in, 8 out]
            n158 = Unbundle By Name(w691) -> ("scriptSelected"=w694:i32)
            n159 = call "runSingleScriptV3.vi"("error in (no error)"=w692, "HWLoop"="HW Loop?", "index"=w694, "ExperimentRunner in"=w691) -> ("error out"=w688:errorcluster, "ExperimentRunner out"=w690:refnum<class "ExperimentRunner.lvclass">)  [unwired: 6 in]
          }
          event "stop": Mouse Down {
            n160 = event-data() -> ()  [unwired: 1 in, 8 out]
            n161 = call "sendStop.vi"("error in (no error)"=w705, "stop"=enum16{"stopBeforeNext", "stopNow"}."stopNow" ("stop 2"), "ExperimentRunner in"=w703) -> ("error out"=w704:errorcluster, "ExperimentRunner out"=w702:refnum<class "ExperimentRunner.lvclass">)  [unwired: 7 in]
          }
          event "staticOutput": Mouse Down {
            n162 = event-data() -> ()  [unwired: 1 in, 8 out]
            n163 = Unbundle By Name(w725) -> ("deviceDataBaseConnection"=w721:refnum<class "deviceDataBase.lvclass">)
            n164 = call "isRunning.vi"("error in (no error)"=w715, "StaticOutputEditor in"=w710) -> ("error out"=w714:errorcluster, "running?"=w713:bool, "StaticOutputEditor out"=w716:refnum<class "StaticOutputEditor.lvclass">)  [unwired: 7 in]
            n165 = case shown="False" w713 {
              tunnel: w724 -> [w737 _]
              tunnel: [w736 w739] -> w723
              tunnel: [w735 w740] -> w722
              tunnel: w721 -> [w734 _]
              tunnel: w716 -> [w730 w741]
              tunnel: w715 -> [w728 w738]
              tunnel: w714 -> [w729 _]
              frame False {
                n166 = call "close.vi"("error in (no error)"=w729, "StaticOutputEditor in"=w730) -> ("error out"=w726:errorcluster, "StaticOutputEditor out"=w727:refnum<class "StaticOutputEditor.lvclass">)  [unwired: 8 in]
                n167 = call "getUnrestrictedChannelArray.vi"("error in (no error)"=w728, "deviceDataBase in"=w734) -> ("error out"=w732:errorcluster, "ChannelArray.lvclass"=w733:refnum<class "ChannelArray.lvclass">)  [unwired: 7 in, 1 out]
                n168 = Merge Errors(w726, w732) -> (w731:errorcluster)
                n169 = call-dynamic "run.vi"("error in (no error)"=w731, "HWControllerEvents"=w737, "ChannelArray"=w733, "StaticOutputEditor"=w727) -> ("error out"=w736:errorcluster, "StaticOutputEditor out"=w735:refnum<class "StaticOutputEditor.lvclass">)  [unwired: 6 in]
              }
              frame True {
                n170 = call "showFrontEnd.vi"("error in (no error)"=w738, "StaticOutputEditor in"=w741) -> ("error out"=w739:errorcluster, "StaticOutputEditor out"=w740:refnum<class "StaticOutputEditor.lvclass">)  [unwired: 8 in]
              }
            }
          }
          event "refreshDatabase": Mouse Down {
            # "close compiler"
            # "Compiler"
            n171 = event-data() -> ()  [unwired: 1 in, 2 out]
            n172 = Unbundle By Name(w765) -> ("deviceDataBaseConnection"=w766:refnum<class "deviceDataBase.lvclass">, "HWControllerEvents"=w751:refnum<class "HWControllerEvents.lvclass">)
            n173 = Bundle(TRUE) -> (w757:cluster{bool})  [unwired: 1 in]
            n174 = Bundle("eventId"=T4."restartCompiler", w757) -> (w756:T17)  [unwired: 1 in]
            n175 = Generate User Event(user event=w759, event data cluster=w756, error in=w753) -> (error out=w752:errorcluster)  [unwired: 1 out]
            n176 = call "loadDatabase.vi"("error in (no error)"=w752, "deviceDataBase in"=w766) -> ("error out"=w749:errorcluster, "deviceDataBase out"=w750:refnum<class "deviceDataBase.lvclass">)  [unwired: 7 in, 1 out]
            n177 = call "close.vi"("error in (no error)"=w749, "Compiler in"=w748) -> ("error out"=w746:errorcluster, "Compiler out"=w747:refnum<class "Compiler.lvclass">)  [unwired: 8 in]
            n178 = call "databaseGF.vi"("deviceDataBase in"=w750, "Enum"=enum16{"write", "read"}."write") -> ()  [unwired: 9 in, 1 out]
            n179 = call "run.vi"("error in (no error)"=w746, "deviceDataBase"=w750, "HWControllerEvents"=w751, "Compiler in"=w747) -> ("error out"=w744:errorcluster, "Compiler out"=w745:refnum<class "Compiler.lvclass">)  [unwired: 6 in]
            n180 = Bundle By Name(cluster=w765, "deviceDataBaseConnection"=w750) -> (w764:refnum<class "ExperimentRunner.lvclass">)
          }
        }
      }
      n181 = call "isRunning.vi"("error in (no error)"=w19, "StaticOutputEditor in"=w21) -> ("error out"=w34:errorcluster, "running?"=w33:bool, "StaticOutputEditor out"=w32:refnum<class "StaticOutputEditor.lvclass">)  [unwired: 7 in]
      n182 = Close Reference(reference=w62, error in (no error)=w19) -> (error out=w52:errorcluster)
      n183 = call "isItRunning.vi"("error in (no error)"=w19, "CameraControlViewer in"=w20) -> ("error out"=w16:errorcluster, "running?"=w18:bool, "CameraControlViewer out"=w17:refnum<class "CameraControlViewer.lvclass">)  [unwired: 7 in]
      n184 = case shown="False" w33 {
        tunnel: w34 -> [w69 w74]
        tunnel: w32 -> [w70 w73]
        tunnel: [w70 w72] -> w31
        tunnel: [w69 w71] -> w30
        frame False {
        }
        frame True {
          n185 = call "showFrontEnd.vi"("error in (no error)"=w74, "StaticOutputEditor in"=w73) -> ("error out"=w71:errorcluster, "StaticOutputEditor out"=w72:refnum<class "StaticOutputEditor.lvclass">)  [unwired: 8 in]
        }
      }
      n186 = case shown="False" w18 {
        tunnel: w17 -> [w64 w68]
        tunnel: w16 -> [w63 w67]
        tunnel: [w64 w66] -> w15
        tunnel: [w63 w65] -> w14
        frame False {
        }
        frame True {
          n187 = call "showFrontEnd.vi"("error in (no error)"=w67, "CameraControlViewer in"=w68) -> ("error out"=w65:errorcluster, "CameraControlViewer out"=w66:refnum<class "CameraControlViewer.lvclass">)  [unwired: 8 in]
        }
      }
      n188 = Close Reference(reference=w53, error in (no error)=w52) -> (error out=w29:errorcluster)
      n189 = call "close.vi"("error in (no error)"=w30, "StaticOutputEditor in"=w31) -> ("error out"=w28:errorcluster)  [unwired: 8 in, 1 out]
      n190 = call "close.vi"("error in (no error)"=w14, "CameraControlViewer in"=w15) -> ("error out"=w13:errorcluster)  [unwired: 8 in, 1 out]
      n191 = call <vilib>:"Clear Errors.vi"("error in (no error)"=w13) -> ("error out"=w12:errorcluster)  [unwired: 6 in]
      n192 = Merge Errors(w29, w12, w28) -> (w50:errorcluster)
    }
    frame Error {
    }
  }
  "error out" <- w9
  "Views.lvlib:ExperimentControl.lvlib:ExperimentRunner out" <- w8
